vi "Front Panel Clean Up.vi"(5 "X_Buffer":u32=20, 7 "Y_Buffer":u32=20, 8 "Error In":errorcluster, 10 "VI Ref":refnum<vi>, 11 "VI Path":path) -> (0 "Error Out":errorcluster={"status"=TRUE, "code"=1026, "source"="Property Node in LVH-Toolbox.lvlib:Move and Resize.vi->LVH-Toolbox.lvlib:Front Panel Clean Up.vi"})   [LabVIEW 2014, in "LMH-Toolbox.lvlib" / "LMH-Front-Panel-Clean-Up.lvlib"]
uses:
  <vilib>/MakerHub/Toolbox/Private/Front Panel Clean Up/LMH-Front-Panel-Clean-Up.lvlib
panel:
  in  "Resize":bool=TRUE
  in  "Reposition":bool=TRUE
  out "Max Heights":string[](array[string])
  out "Max Widths":u32[](array[numeric])
  out "Connector Pane":string[][](array[string])
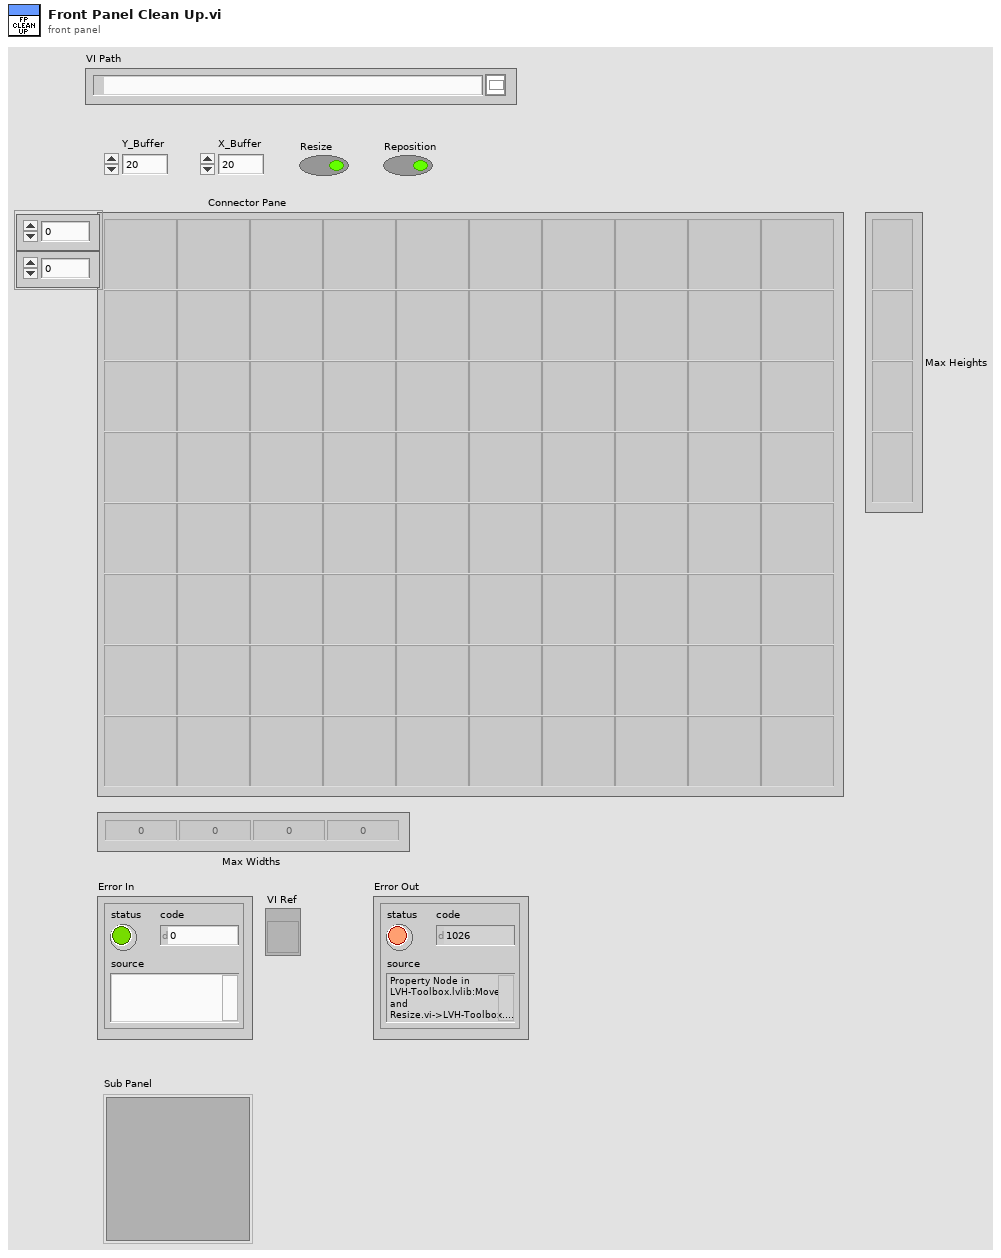
[diagram p1: front panel]
types:
  T1 = typedef "LMH-Toolbox.lvlib/LMH-Front-Panel-Clean-Up.lvlib/FP Data.ctl" = cluster{"VI Ref":refnum<vi>, "FP Objects":refnum<vi>[][], "FP Object Names":string[][], "Max Widths":u32[], "Max Heights":u32[]}
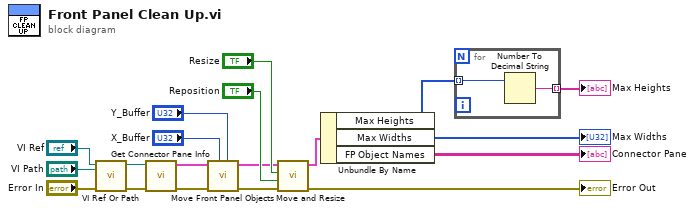
[diagram p0: block diagram]
diagram:
  n1 = call <vilib>:"VI Ref Or Path.vi"("Error In"="Error In", "VI Path"="VI Path", "VI Ref"="VI Ref") -> ("Error Out"=w14:errorcluster, "VI out"=w15:refnum<vi>)  [unwired: 7 in]
  n2 = call <vilib>:"Get Connector Pane Info.vi"("Error In"=w14, "VI Ref"=w15) -> ("Error Out"=w19:errorcluster, "FP Data"=w12:T1)  [unwired: 8 in]
  n3 = call <vilib>:"Move Front Panel Objects.vi"("Y_Buffer"="Y_Buffer", "X_Buffer"="X_Buffer", "Error In"=w19, "FP Data"=w12) -> ("Error Out"=w10:errorcluster, "FP Data"=w3:T1)  [unwired: 6 in]
  n4 = call <vilib>:"Move and Resize.vi"("Error In"=w10, "Reposition"="Reposition", "Resize"="Resize", "FP Data"=w3) -> ("Error Out"=→"Error Out":errorcluster, "FP Data"=w2:T1)  [unwired: 6 in]
  n5 = Unbundle By Name(w2) -> ("Max Heights"=w6:u32[], "Max Widths"=→"Max Widths":u32[], "FP Object Names"=→"Connector Pane":string[][])
  n6 = for {
    tunnel: [w21] -> w18 mode=indexing
    tunnel: w6 -> [w20] mode=indexing
    n7 = Number To Decimal String(number=w20) -> (decimal integer string=w21:string)  [unwired: 1 in]
  }
  "Max Heights" <- w18
